vi "Read Elavator Location.vi"(8 "error in (no error)":errorcluster, 11 "Display Console in":refnum<class "Display Console.lvclass">) -> (0 "error out":errorcluster, 2 "Elevator Position":string, 3 "Display Console out":refnum<class "Display Console.lvclass">)   [LabVIEW 2019, in "Display Console Actor.lvlib" / "Display Console.lvclass"]
uses:
  Display Console.lvclass
  Display Console.lvclass/Display Console.ctl
  Abstract Display Console Actor/Abstract Display Console Actor/Abstract Display Console.lvclass
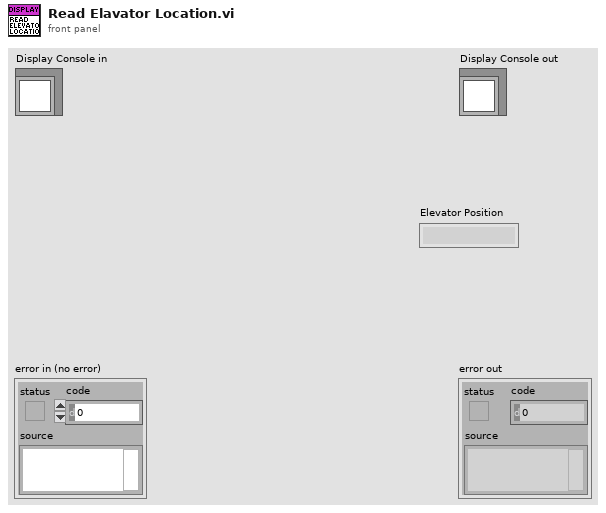
[diagram p1: front panel]
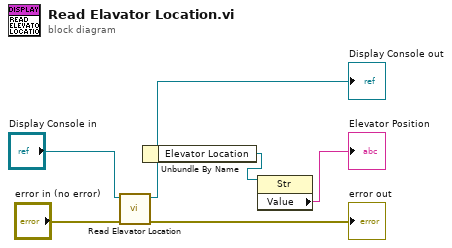
[diagram p0: block diagram]
diagram:
  n1 = call-parent "Read Elavator Location.vi"("error in (no error)"="error in (no error)", "Abstract Display Console in"="Display Console in") -> ("error out"=→"error out":errorcluster, "Abstract Display Console out"=w3:refnum<class "Display Console.lvclass">)  [unwired: 7 in, 1 out]
  "Display Console out" <- w3
  n2 = Unbundle By Name(w3) -> ("Elevator Location"=w2:refnum<vi>)
  n3 = property class="Str"(reference=w2) -> ("Value"=→"Elevator Position":string)  [unwired: 1 in, 2 out]
